vi "SimulatoreStep.vi"() -> ()   [LabVIEW 2019]
doc: "Simulatore Step dei Test:\n\n1. Seleziona la postazione con la data di partenza (opzionale)\n2. Seleziona il Test che vuoi eseguire\n3. Avvia la simulazione e verifica il successo degli Step"
uses:
  ByteGSAPIBase/ByteGSAPIBase.lvclass
  TypeDef/StepSimulationInfo.ctl
  TypeDef/ProcessStatus.ctl
  TypeDef/SimulatoreStates.ctl
  ByteGSAPIBase/TypeDef/Step.ctl
  ByteGSAPIBase/TypeDef/Asset.ctl
  ByteGSAPIBase/TypeDef/Test.ctl
  <vilib>/numeric/Random Number (Range) U64.vi
  <vilib>/numeric/sub_Random U32.vi
panel:
  out "Title":string
  out "Status Control":T2
  out "Waveform Chart":cluster{"Time Elapsed":dbl, dbl}(graph)
  out "Step Info List":T3[](array[typedef])
  in  "Step simulation":bool
  out "Infos":string
  in  "Inizia Test":bool
  in  "Select Test":i32(ring) items=["T0014 - Endurance test"=54, "T0011 - Endurance test 19/02/2025"=51, "T0010 - Endurance test 19/02/2025"=50, "T0009 - Endurance test 19/02/2025"=49, "T0006 - Endurance Test"=46, "T0007 - Endurance Test"=47, "T0012 - Endurance test"=52, "T0013 - Endurance test"=53, "T0005 - Endurance Test"=45, "T0015 - Endurance test"=55, "T0008 - Endurance test 19/02/2025"=48, "T0016 - Endurance test"=56]
  in  "ByteGSAPIBase in":refnum<class "ByteGSAPIBase.lvclass">
  in  "Exit":bool
  in  "Home":bool
  in  "Ottieni Test Per Postazione":bool
  in  "Starting Date":timestamp format="%<%x>T"
  in  "Workstation":u16(ring) items=["Sala gialla", "POST 1"]
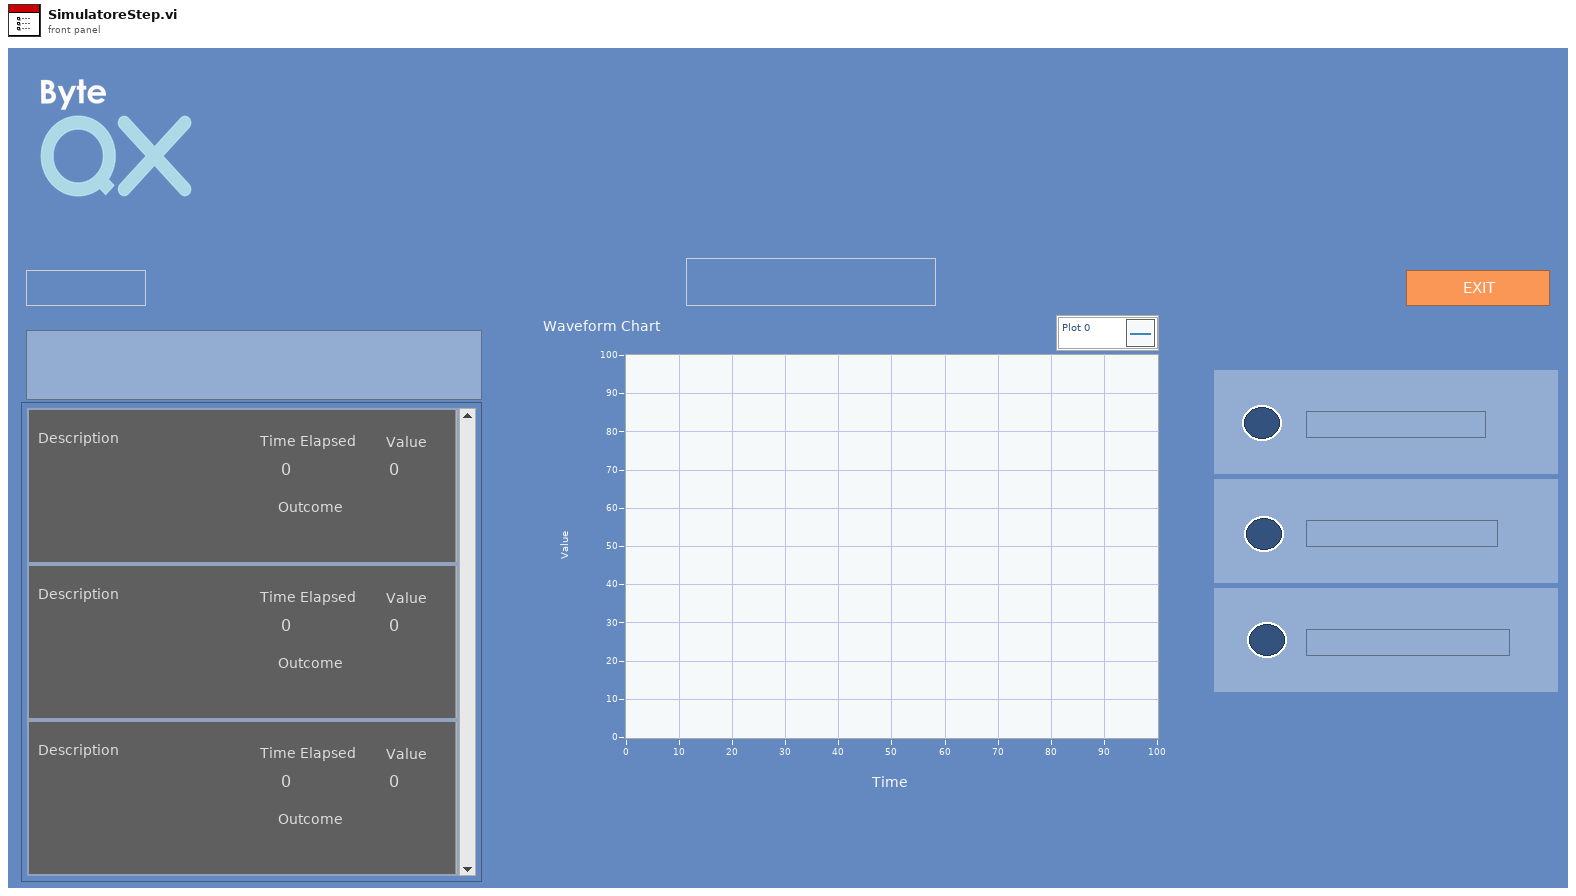
[diagram p1: front panel]
types:
  T1 = typedef "ProcessStatus.ctl" = cluster{"Active":bool, "Process":string}
  T2 = cluster{"Cluster":T1, "Cluster 2":T1, "Cluster 3":T1}
  T3 = typedef "StepSimulationInfo.ctl" = cluster{"Description":string, "Value":dbl, "Outcome":string, "Time Elapsed":dbl, "id":dbl, "Color Box":u32}
  T4 = typedef "SimulatoreStates.ctl" = enum16{"Initialize", "Idle", "GetLimsTestsForBench", "GetLimsTestSteps", "Simulation Start", "WaitForLigths"}
  T5 = typedef "ByteQXWebAPI.lvlib/ByteGSAPIBase.lvclass/Test.ctl" = cluster{"titolo":string, "descrizione":string, "statoprova":string, "assets":T6[], "id":i32, "data_apertura_prova":timestamp, "slug":string}
  T6 = typedef "ByteQXWebAPI.lvlib/ByteGSAPIBase.lvclass/Asset.ctl" = cluster{"descrizione":string, "slug":string, "id":i32}
  T7 = typedef "ByteQXWebAPI.lvlib/ByteGSAPIBase.lvclass/Step.ctl" = cluster{"id":i32, "descrizione":string, "prova":cluster{"slug":string}, "assets":T6[], "criterio_accettazione":string, "valore_criterio_accettazione_max":dbl, "valore_criterio_accettazione_min":dbl, "udm_criterio_accettazione":string, "duration_prova":string, "udm_duration_prova":string, "valore_prova":dbl, "ordine":i32, "user":i32, "link_automation":string, "instruction_automation":string, "data_completamento_checklist":timestamp, "outcome":bool, "step_type":string, "channels":string[]}
  T8 = cluster{"ByteGSAPIBase in":refnum<class "ByteGSAPIBase.lvclass">, "Array dei Test":T5[], "Steps Array":T7[], "Step Info List":T3[], "index":i32, "Previus":T4, "Infos":string, "State":T4, "Status Control":cluster{"Cluster":T1, "Cluster 2":T1, "Cluster 3":T1}, "light position":i32}
  T9 = cluster{"Workstation":refnum<vi>, "Starting Date":refnum<vi>, "Ottieni Test Per Postazione":refnum<vi>, "Infos":refnum<vi>, "Inizia Test":refnum<vi>, "Select Test":refnum<vi>, "Step Info List":refnum<vi>, "Step simulation":refnum<vi>, "Waveform Chart":refnum<vi>, "Status Control":refnum<vi>, "Title":refnum<vi>}
  T10 = enum8{"Enabled", "Disabled", "Disabled and Grayed Out"}
  T11 = cluster{"Workstation":u16, "Starting Date":timestamp, "Select Test":i32}
  T12 = typedef "ByteQXWebAPI.lvlib/ByteGSAPIBase.lvclass/UpdateLimsTestStepData.ctl" = cluster{"outcome":bool, "data_completamento_checklist":timestamp, "udm_duration_prova":string, "valore_prova":dbl, "link_automation":string, "instruction_automation":string, "duration_prova":string}
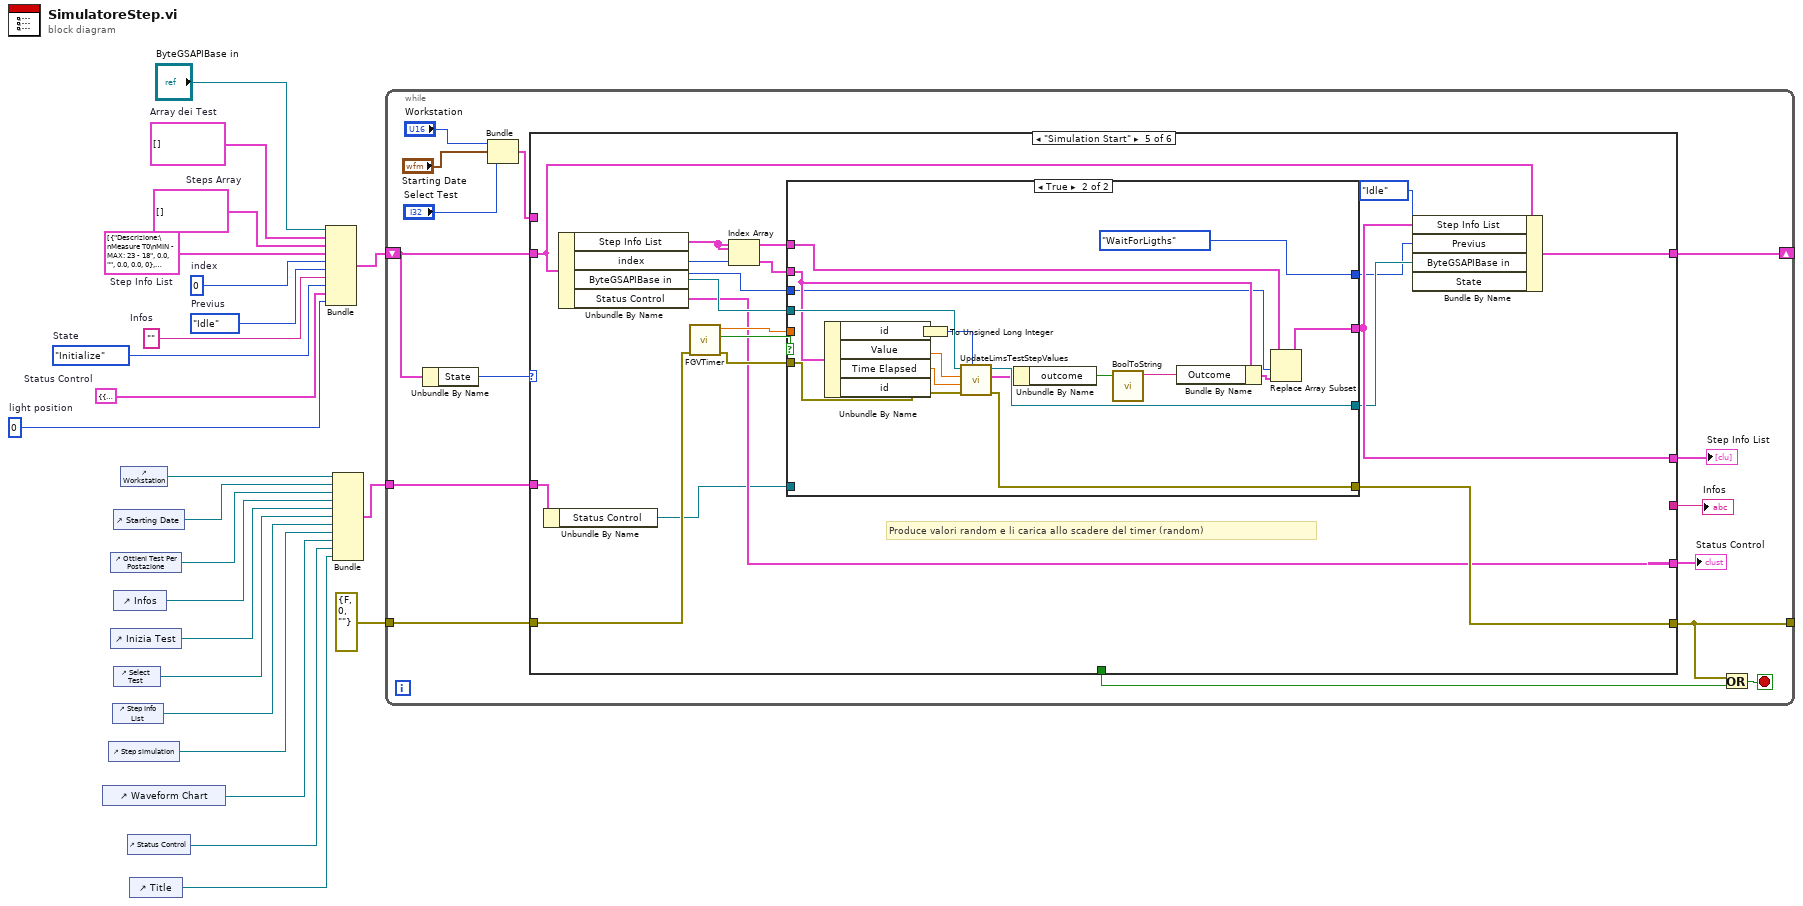
[diagram p0: block diagram]
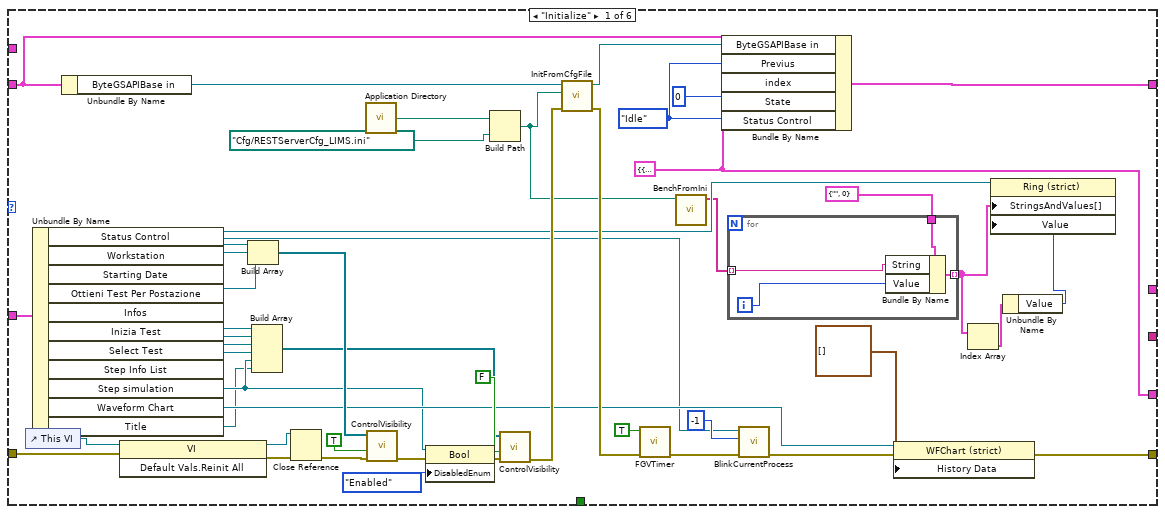
[diagram p2: hidden frame]
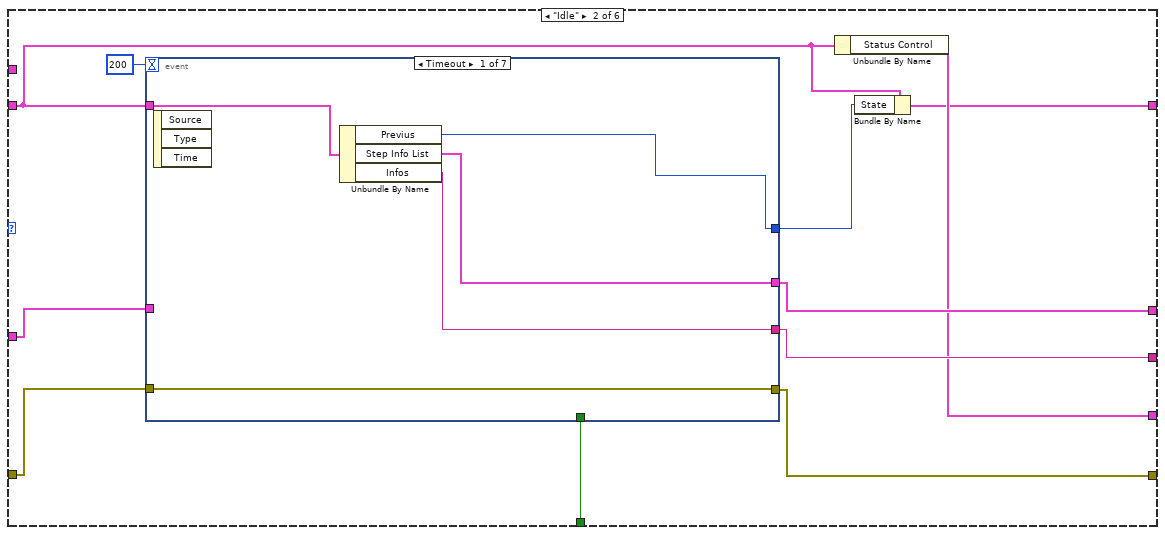
[diagram p3: hidden frame]
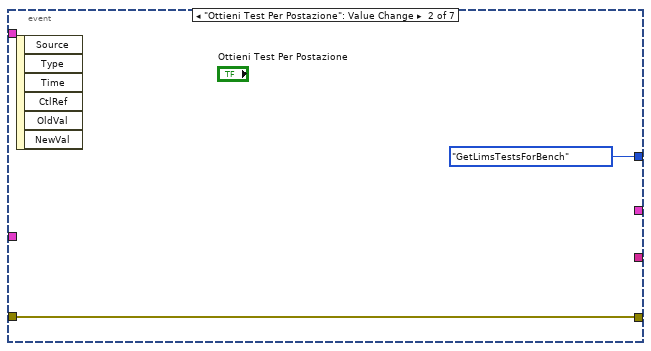
[diagram p4: hidden frame]
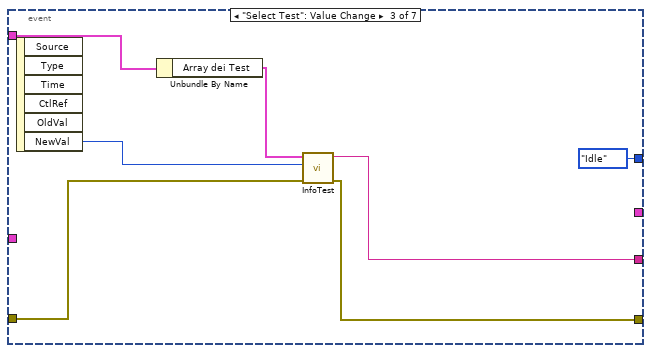
[diagram p5: hidden frame]
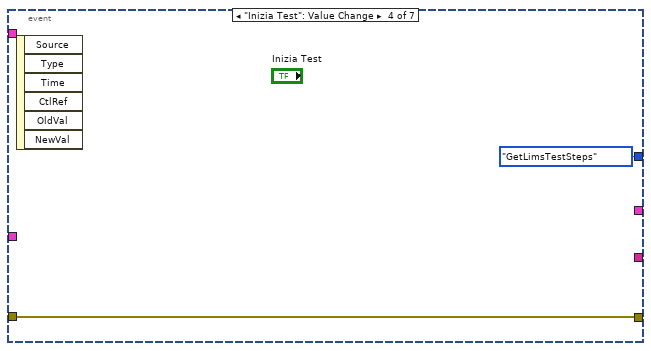
[diagram p6: hidden frame]
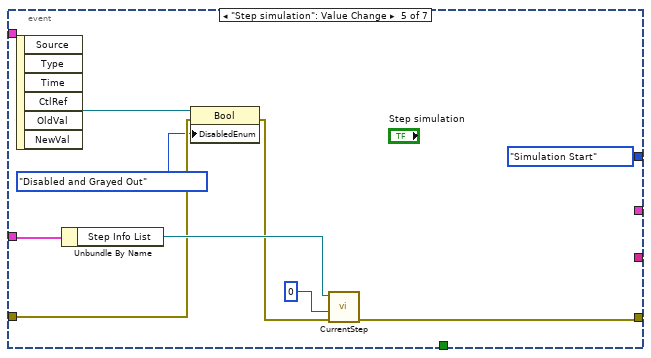
[diagram p7: hidden frame]
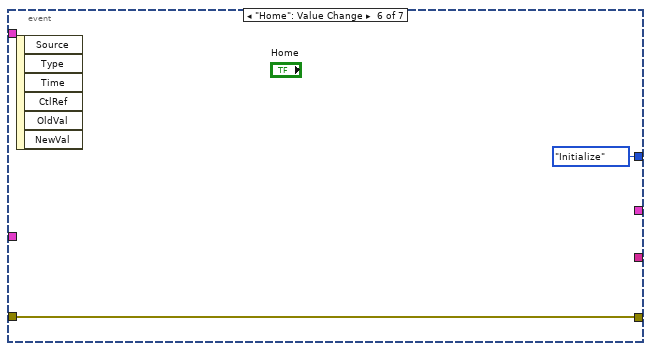
[diagram p8: hidden frame]
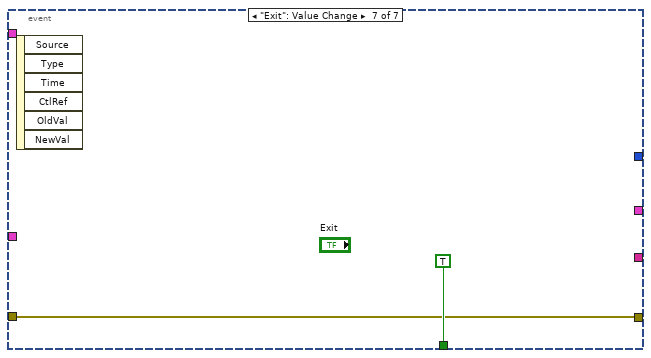
[diagram p9: hidden frame]
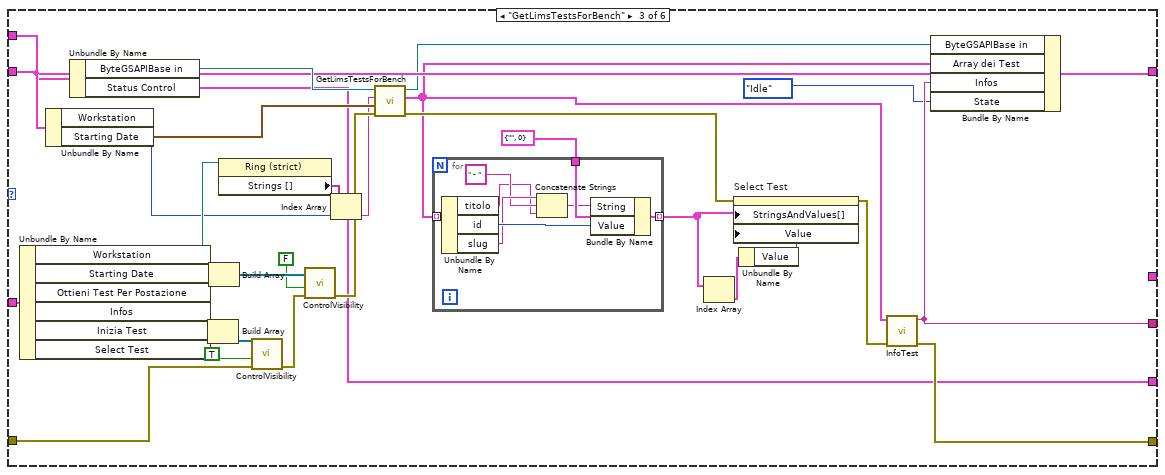
[diagram p10: hidden frame]
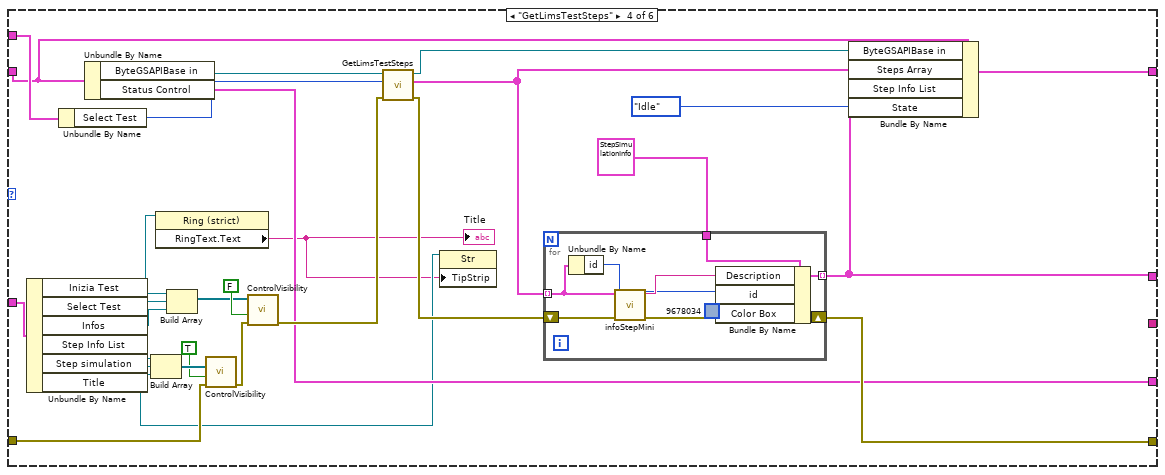
[diagram p11: hidden frame]
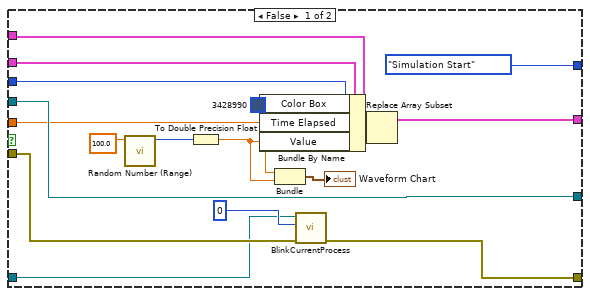
[diagram p12: hidden frame]
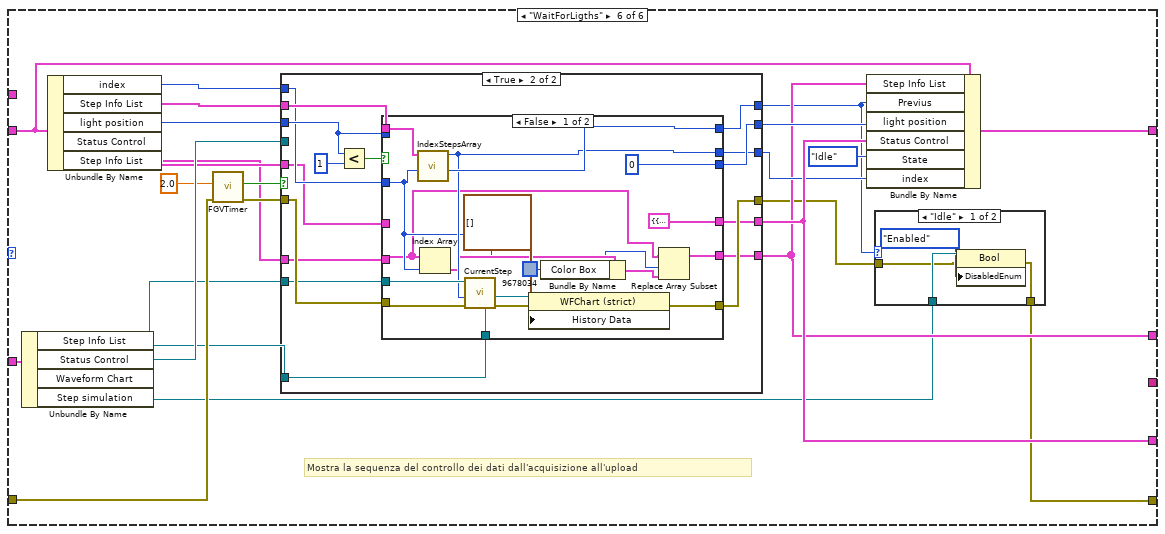
[diagram p13: hidden frame]
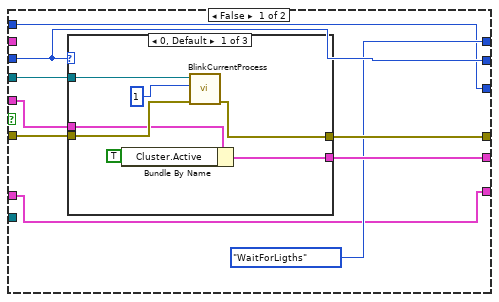
[diagram p15: hidden frame]
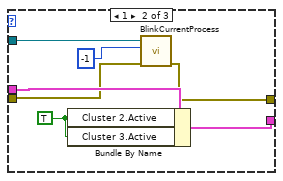
[diagram p16: hidden frame]
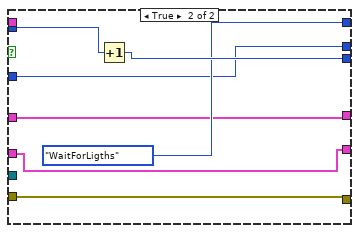
[diagram p18: hidden frame]
diagram:
  w5 = 0  # light position
  w6 = T2 {"Cluster"={"Active"=FALSE, "Process"="Acquisizione Dati"}, "Cluster 2"={"Active"=FALSE, "Process"="Upload Dati"}, "Cluster 3"={"Active"=FALSE, "Process"="Upload Completato"}}  # Status Control
  w9 = ""  # Infos
  w10 = SimulatoreStates."Idle"  # Previus
  w11 = 0  # index
  w12 = T3[] [{"Description"="Descrizione:\nMeasure T0\nMIN - MAX: 23 - 18", "Value"=0.0, "Outcome"="", "Time Elapsed"=0.0, "id"=0.0, "Color Box"=0}, {"Description"="Descrizione:\nSet Nominsl Torque\nMIN - MAX: 1 - -1", "Value"=0.0, "Outcome"="", "Time Elapsed"=0.0, "id"=0.0, "Color Box"=0}, {"Description"="Descrizione:\nVibrazione X,Y,Z\nMIN - MAX: 0 - 0", "Value"=0.0, "Outcome"="", "Time Elapsed"=0.0, "id"=0.0, "Color Box"=0}, {"Description"="Descrizione:\nPlace Motor on the bench. Plug wires on terminal block.\nMIN - MAX: 0 - 0", "Value"=0.0, "Outcome"="", "Time Elapsed"=0.0, "id"=0.0, "Color Box"=0}, {"Description"="Descrizione:\nMeasure R01\nMIN - MAX: 0 - 0", "Value"=0.0, "Outcome"="", "Time Elapsed"=0.0, "id"=0.0, "Color Box"=0}, {"Description"="Descrizione:\nMeasure R02\nMIN - MAX: 0 - 0", "Value"=0.0, "Outcome"="", "Time Elapsed"=0.0, "id"=0.0, "Color Box"=0}]  # Step Info List
  w19 = T5[] []  # Array dei Test
  w18 = T7[] []  # Steps Array
  w8 = SimulatoreStates."Initialize"  # State
  n1 = control-ref of="Waveform Chart"() -> (w3:refnum<vi>)
  n2 = control-ref of="Step simulation"() -> (w13:refnum<vi>)
  n3 = control-ref of="Ottieni Test Per Postazione"() -> (w22:refnum<vi>)
  n4 = control-ref of="Inizia Test"() -> (w15:refnum<vi>)
  n5 = control-ref of="Step Info List"() -> (w4:refnum<vi>)
  n6 = control-ref of="Starting Date"() -> (w23:refnum<vi>)
  n7 = control-ref of="Infos"() -> (w16:refnum<vi>)
  n8 = control-ref of="Select Test"() -> (w14:refnum<vi>)
  n9 = control-ref of="Workstation"() -> (w24:refnum<vi>)
  n10 = control-ref of="Status Control"() -> (w2:refnum<vi>)
  n11 = control-ref of="Title"() -> (w1:refnum<vi>)
  n12 = Bundle("ByteGSAPIBase in"="ByteGSAPIBase in", "Array dei Test"=w19, "Steps Array"=w18, "Step Info List"=w12, "index"=w11, "Previus"=w10, "Infos"=w9, "State"=w8, "Status Control"=w6, "light position"=w5) -> (w17:T8)  [unwired: 1 in]
  n13 = Bundle("Workstation"=w24, "Starting Date"=w23, "Ottieni Test Per Postazione"=w22, "Infos"=w16, "Inizia Test"=w15, "Select Test"=w14, "Step Info List"=w4, "Step simulation"=w13, "Waveform Chart"=w3, "Status Control"=w2, "Title"=w1) -> (w21:T9)  [unwired: 1 in]
  n14 = while {
    tunnel: w21 -> [w35]
    shift-right: [w34] -> _
    shift-left: w17 -> [w28]
    tunnel: errorcluster {"status"=FALSE, "code"=0, "source"=""} ("error in (no error)") -> [w39]
    tunnel: [w31] -> _
    stop <- w30 stop-if-true
    n15 = Unbundle By Name(w28) -> ("State"=w27:T4)
    n16 = Bundle("Workstation"="Workstation", "Starting Date"="Starting Date", "Select Test"="Select Test") -> (w36:T11)  [unwired: 1 in]
    n17 = case shown="\"Simulation Start\"" w27 {
      tunnel: w39 -> [w85 w101 w158 w184 w225 w280]
      tunnel: w36 -> [_ _ w163 w200 _ _]
      tunnel: w35 -> [w82 w95 w154 w194 w212 w282]
      tunnel: [w60 w99 w145 w188 w214 w262] -> w31
      tunnel: w28 -> [w73 w92 w162 w197 w222 w277]
      tunnel: [w72 w91 w160 w196 w218 w276] -> w34
      tunnel: [_ w100 w140 _ _ _] -> w32
      tunnel: [_ w97 _ w180 w219 w266] -> w26
      tunnel: [_ w96 _ _ _ _] -> w29
      tunnel: [w54 w93 w137 w177 w210 w274] -> w25
      frame "Initialize" {
        w54 = T2 {"Cluster"={"Active"=FALSE, "Process"="DATA AQUISITION"}, "Cluster 2"={"Active"=FALSE, "Process"="DATA UPLOAD"}, "Cluster 3"={"Active"=FALSE, "Process"="LOADING NEXT STEP"}} ("Status Control")
        w61 = SimulatoreStates."Idle"
        n18 = control-ref of="This VI"() -> (w86:refnum<vi>)
        n19 = Unbundle By Name(w82) -> ("Status Control"=w53:refnum<vi>, "Workstation"=w45:refnum<vi>, "Starting Date"=w81:refnum<vi>, "Ottieni Test Per Postazione"=w80:refnum<vi>, "Infos"=w69:refnum<vi>, "Inizia Test"=w68:refnum<vi>, "Select Test"=w67:refnum<vi>, "Step Info List"=w65:refnum<vi>, "Step simulation"=w50:refnum<vi>, "Waveform Chart"=w59:refnum<vi>, "Title"=w48:refnum<vi>)
        n20 = Unbundle By Name(w73) -> ("ByteGSAPIBase in"=w74:refnum<class "ByteGSAPIBase.lvclass">)
        n21 = invoke class="VI" method="Default Vals.Reinit All"(reference=w86, error in=w85) -> (reference out=w84:refnum<vi>, error out=w83:errorcluster)  [unwired: 1 in, 1 out]
        n22 = Build Array(w45, w81, w80) -> (w79:refnum<vi>[])
        n23 = Build Array(w69, w68, w67, w65, w50, w48) -> (w66:refnum<vi>[])
        n24 = Close Reference(reference=w84, error in (no error)=w83) -> (error out=w78:errorcluster)
        n25 = call <vilib>:"Application Directory.vi"() -> ("Application Directory"=w76:path)
        n26 = call "ControlVisibility.vi"("error in (no error)"=w78, "Visible"=TRUE, "Controls"=w79) -> ("error out"=w52:errorcluster)  [unwired: 8 in]
        n27 = property class="Bool"(reference=w50, error in=w52, "DisabledEnum"=T10."Enabled" ("Disabled")) -> (error out=w51:errorcluster)  [unwired: 1 out]
        n28 = Build Path(base path=w76, name or relative path=path "Cfg/RESTServerCfg_LIMS.ini") -> (appended path=w46:path)
        n29 = call "ControlVisibility.vi"("error in (no error)"=w51, "Visible"=FALSE, "Controls"=w66) -> ("error out"=w71:errorcluster)  [unwired: 8 in]
        n30 = call-dynamic "InitFromCfgFile.vi"("error in (no error)"=w71, "configuration file path"=w46, "ByteGSAPIBase in"=w74) -> ("error out"=w64:errorcluster, "ByteGSAPIBase out"=w75:refnum<class "ByteGSAPIBase.lvclass">)  [unwired: 7 in]
        n31 = call "FGVTimer.vi"("error in"=w64, "Reset"=TRUE) -> ("error out"=w57:errorcluster)  [unwired: 7 in, 2 out]
        n32 = call "BenchFromIni.vi"("configuration file path"=w46) -> ("Array"=w44:string[])  [unwired: 9 in, 1 out]
        n33 = Bundle By Name(cluster=w73, "ByteGSAPIBase in"=w75, "Previus"=w61, "index"=0, "State"=w61, "Status Control"=w54) -> (w72:T8)
        n34 = for {
          tunnel: [w90] -> w41 mode=indexing
          tunnel: w44 -> [w89] mode=indexing
          tunnel: cluster{"String":string, "Value":u16} {"String"="", "Value"=0} ("Cluster") -> [w87]
          i -> [w88]
          n35 = Bundle By Name(cluster=w87, "String"=w89, "Value"=w88) -> (w90:cluster{"String":string, "Value":u16})
        }
        n36 = call "BlinkCurrentProcess.vi"("error in (no error)"=w57, "index"=-1, "Status Control"=w53) -> ("error out"=w56:errorcluster)  [unwired: 8 in]
        n37 = property class="WFChart (strict)"(reference=w59, error in=w56, "History Data"=cluster{"Time Elapsed":dbl, dbl}[] []) -> (error out=w60:errorcluster)  [unwired: 1 out]
        n38 = Index Array(array=w41) -> (element=w42:cluster{"String":string, "Value":u16})  [unwired: 1 in]
        n39 = Unbundle By Name(w42) -> ("Value"=w40:u16)
        n40 = property class="Ring (strict)"(reference=w45, "StringsAndValues[]"=w41, "Value"=w40) -> ()  [unwired: 1 in, 2 out]
      }
      frame "Idle" {
        n41 = event shown="[0] Timeout" {
          selector: _ -> [_ _ _ _ _ _ _]
          dyn-events: _ -> [_ _ _ _ _ _ _]
          timeout: 200 -> [_ _ _ _ _ _ _]
          tunnel: [w102 SimulatoreStates."GetLimsTestsForBench" SimulatoreStates."Idle" SimulatoreStates."GetLimsTestSteps" SimulatoreStates."Simulation Start" SimulatoreStates."Initialize" _] -> w94
          tunnel: [w104 _ w114 _ _ _ _] -> w100
          tunnel: w101 -> [w103 w107 w113 w116 w120 w127 w129]
          tunnel: [w103 w107 w112 w116 w124 w127 w129] -> w99
          tunnel: w92 -> [w106 _ w111 _ _ _ _]
          tunnel: [w105 _ _ _ _ _ _] -> w97
          tunnel: [_ _ _ _ _ _ TRUE] -> w96
          tunnel: w95 -> [_ _ _ _ w125 _ _]
          event Timeout {
            n42 = event-data() -> ()  [unwired: 1 in, 3 out]
            n43 = Unbundle By Name(w106) -> ("Previus"=w102:T4, "Step Info List"=w105:T3[], "Infos"=w104:string)
          }
          event "Ottieni Test Per Postazione": Value Change {
            n44 = event-data() -> ()  [unwired: 1 in, 6 out]
          }
          event "Select Test": Value Change {
            n45 = event-data() -> ("NewVal"=w110:i32)  [unwired: 1 in, 5 out]
            n46 = Unbundle By Name(w111) -> ("Array dei Test"=w109:T5[])
            n47 = call "InfoTest.vi"("error in"=w113, "Seleziona Test"=w110, "TestForBenchArray"=w109) -> ("error out"=w112:errorcluster, "Info Test"=w114:string)  [unwired: 7 in]
          }
          event "Inizia Test": Value Change {
            n48 = event-data() -> ()  [unwired: 1 in, 6 out]
          }
          event "Step simulation": Value Change {
            n49 = event-data() -> ("CtlRef"=w121:refnum<vi>)  [unwired: 1 in, 5 out]
            n50 = Unbundle By Name(w125) -> ("Step Info List"=w122:refnum<vi>)
            n51 = property class="Bool"(reference=w121, error in=w120, "DisabledEnum"=T10."Disabled and Grayed Out" ("Disabled")) -> (error out=w119:errorcluster)  [unwired: 1 out]
            n52 = call "CurrentStep.vi"("error in (no error)"=w119, "index"=0, "Array in"=w122) -> ("error out"=w124:errorcluster)  [unwired: 8 in]
          }
          event "Home": Value Change {
            n53 = event-data() -> ()  [unwired: 1 in, 6 out]
          }
          event "Exit": Value Change {
            n54 = event-data() -> ()  [unwired: 1 in, 6 out]
          }
        }
        n55 = Unbundle By Name(w92) -> ("Status Control"=w93:T2)
        n56 = Bundle By Name(cluster=w92, "State"=w94) -> (w91:T8)
      }
      frame "GetLimsTestsForBench" {
        n57 = Unbundle By Name(w154) -> ("Workstation"=w134:refnum<vi>, "Starting Date"=w153:refnum<vi>, "Ottieni Test Per Postazione"=w152:refnum<vi>, "Infos"=w151:refnum<vi>, "Inizia Test"=w150:refnum<vi>, "Select Test"=w149:refnum<vi>)
        n58 = Unbundle By Name(w163) -> ("Workstation"=w132:u16, "Starting Date"=w139:timestamp)
        n59 = Unbundle By Name(w162) -> ("ByteGSAPIBase in"=w164:refnum<class "ByteGSAPIBase.lvclass">, "Status Control"=w137:T2)
        n60 = Build Array(w151, w150, w149) -> (w143:refnum<vi>[])
        n61 = Build Array(w134, w153, w152) -> (w144:refnum<vi>[])
        n62 = property class="Ring (strict)"(reference=w134) -> ("Strings []"=w133:string[])  [unwired: 1 in, 2 out]
        n63 = call "ControlVisibility.vi"("error in (no error)"=w158, "Visible"=TRUE, "Controls"=w143) -> ("error out"=w148:errorcluster)  [unwired: 8 in]
        n64 = call "ControlVisibility.vi"("error in (no error)"=w148, "Visible"=FALSE, "Controls"=w144) -> ("error out"=w147:errorcluster)  [unwired: 8 in]
        n65 = Index Array(array=w133, index=w132) -> (element=w131:string)
        n66 = call-dynamic "GetLimsTestsForBench.vi"("error in (no error)"=w147, "creation date"=w139, "workbench"=w131, "ByteGSAPIBase in"=w164) -> ("error out"=w136:errorcluster, "list of tests"=w135:T5[], "ByteGSAPIBase out"=w161:refnum<class "ByteGSAPIBase.lvclass">)  [unwired: 5 in]
        n67 = for {
          tunnel: [w171] -> w157 mode=indexing
          tunnel: cluster{"String":string, "Value":u16} {"String"="", "Value"=0} ("Cluster") -> [w170]
          tunnel: w135 -> [w169] mode=indexing
          n68 = Unbundle By Name(w169) -> ("titolo"=w166:string, "id"=w172:i32, "slug"=w168:string)
          n69 = Concatenate Strings(w168, " - " ("string"), w166) -> (w165:string)
          n70 = Bundle By Name(cluster=w170, "String"=w165, "Value"=w172) -> (w171:cluster{"String":string, "Value":u16})
        }
        n71 = Index Array(array=w157) -> (element=w156:cluster{"String":string, "Value":u16})  [unwired: 1 in]
        n72 = Unbundle By Name(w156) -> ("Value"=w155:u16)
        n73 = property on="Select Test" class="Ring (strict)"(error in=w136, "StringsAndValues[]"=w157, "Value"=w155) -> (error out=w146:errorcluster)  [unwired: 1 in, 1 out]
        n74 = call "InfoTest.vi"("error in"=w146, "TestForBenchArray"=w135) -> ("error out"=w145:errorcluster, "Info Test"=w140:string)  [unwired: 8 in]
        n75 = Bundle By Name(cluster=w162, "ByteGSAPIBase in"=w161, "Array dei Test"=w135, "Infos"=w140, "State"=SimulatoreStates."Idle") -> (w160:T8)
      }
      frame "GetLimsTestSteps" {
        n76 = Unbundle By Name(w194) -> ("Inizia Test"=w193:refnum<vi>, "Select Test"=w176:refnum<vi>, "Infos"=w187:refnum<vi>, "Step Info List"=w186:refnum<vi>, "Step simulation"=w181:refnum<vi>, "Title"=w174:refnum<vi>)
        n77 = Unbundle By Name(w200) -> ("Select Test"=w175:i32)
        n78 = Unbundle By Name(w197) -> ("ByteGSAPIBase in"=w199:refnum<class "ByteGSAPIBase.lvclass">, "Status Control"=w177:T2)
        n79 = Build Array(w186, w181, w174) -> (w185:refnum<vi>[])
        n80 = property class="Ring (strict)"(reference=w176) -> ("RingText.Text"=w173:string)  [unwired: 1 in, 2 out]
        "Title" <- w173
        n81 = Build Array(w193, w176, w187) -> (w192:refnum<vi>[])
        n82 = call "ControlVisibility.vi"("error in (no error)"=w184, "Visible"=TRUE, "Controls"=w185) -> ("error out"=w183:errorcluster)  [unwired: 8 in]
        n83 = call "ControlVisibility.vi"("error in (no error)"=w183, "Visible"=FALSE, "Controls"=w192) -> ("error out"=w191:errorcluster)  [unwired: 8 in]
        n84 = call-dynamic "GetLimsTestSteps.vi"("error in (no error)"=w191, "test-id"=w175, "ByteGSAPIBase in"=w199) -> ("error out"=w189:errorcluster, "list of steps"=w190:T7[], "ByteGSAPIBase out"=w198:refnum<class "ByteGSAPIBase.lvclass">)  [unwired: 6 in]
        n85 = property class="Str"(reference=w174, "TipStrip"=w173) -> ()  [unwired: 1 in, 2 out]
        n86 = for {
          tunnel: w190 -> [w203] mode=indexing
          shift-right: [w207] -> w188
          shift-left: w189 -> [w208]
          tunnel: T3 {"Description"="Descrizione:\nMeasure T0\nMIN - MAX: 23 - 18", "Value"=0.0, "Outcome"="", "Time Elapsed"=0.0, "id"=0.0, "Color Box"=0} ("Cluster") -> [w206]
          tunnel: [w204] -> w180 mode=indexing
          n87 = Unbundle By Name(w203) -> ("id"=w202:i32)
          n88 = call "infoStepMini.vi"("error in (no error)"=w208, "StepList"=w203) -> ("error out"=w207:errorcluster, "Info Test"=w205:string)  [unwired: 8 in]
          n89 = Bundle By Name(cluster=w206, "Description"=w205, "id"=w202, "Color Box"=u32 9678034) -> (w204:T3)
        }
        n90 = Bundle By Name(cluster=w197, "ByteGSAPIBase in"=w198, "Steps Array"=w190, "Step Info List"=w180, "State"=SimulatoreStates."Idle") -> (w196:T8)
      }
      frame "Simulation Start" {
        # "Produce valori random e li carica allo scadere del timer (random)"
        n91 = Unbundle By Name(w212) -> ("Status Control"=w209:refnum<vi>)
        n92 = Unbundle By Name(w222) -> ("Step Info List"=w221:T3[], "index"=w220:i32, "ByteGSAPIBase in"=w217:refnum<class "ByteGSAPIBase.lvclass">, "Status Control"=w210:T2)
        n93 = call "FGVTimer.vi"("error in"=w225) -> ("error out"=w216:errorcluster, "Elapsed?"=w226:bool, "Time Elapsed"=w223:dbl)  [unwired: 8 in]
        n94 = Index Array(array=w221, index=w220) -> (element=w224:T3)
        n95 = case shown="True" w226 {
          tunnel: w224 -> [w243 w257]
          tunnel: w223 -> [w234 _]
          tunnel: w221 -> [w241 w251]
          tunnel: w220 -> [w235 w252]
          tunnel: [w239 w260] -> w219
          tunnel: w217 -> [w238 w258]
          tunnel: w216 -> [w232 w248]
          tunnel: [w238 w254] -> w215
          tunnel: [w231 w246] -> w214
          tunnel: [SimulatoreStates."Simulation Start" ("Previus") SimulatoreStates."WaitForLigths" ("Previus")] -> w213
          tunnel: w209 -> [w227 _]
          frame False {
            n96 = call-poly <vilib>:"Random Number (Range).vi"("upper bound (100)"=100.0) -> ("number"=w236:u64)  [unwired: 10 in]
            n97 = To Double Precision Float(number=w236) -> (double precision float=w233:dbl)
            n98 = Bundle By Name(cluster=w243, "Color Box"=u32 3428990, "Time Elapsed"=w234, "Value"=w233) -> (w240:T3)
            n99 = Bundle("Time Elapsed"=w234, w233) -> (→"Waveform Chart":cluster{"Time Elapsed":dbl, dbl})  [unwired: 1 in]
            n100 = call "BlinkCurrentProcess.vi"("error in (no error)"=w232, "index"=0, "Status Control"=w227) -> ("error out"=w231:errorcluster)  [unwired: 8 in]
            n101 = Replace Array Subset(array=w241, new element=w240, index=w235) -> (w239:T3[])
          }
          frame True {
            n102 = Unbundle By Name(w257) -> ("id"=w245:dbl, "Value"=w256:dbl, "Time Elapsed"=w255:dbl)  [unwired: 1 out]
            n103 = To Unsigned Long Integer(number=w245) -> (unsigned 32bit integer=w244:u32)
            n104 = call-dynamic "UpdateLimsTestStepValues.vi"("step-id"=w244, "error in (no error)"=w248, "duration hours"=w255, "value"=w256, "ByteGSAPIBase in"=w258) -> ("error out"=w246:errorcluster, "step result"=w253:T12, "ByteGSAPIBase out"=w254:refnum<class "ByteGSAPIBase.lvclass">)  [unwired: 4 in]
            n105 = Unbundle By Name(w253) -> ("outcome"=w249:bool)
            n106 = call "BoolToString.vi"("outcome"=w249) -> ("String"=w250:string)  [unwired: 10 in]
            n107 = Bundle By Name(cluster=w257, "Outcome"=w250) -> (w259:T3)
            n108 = Replace Array Subset(array=w251, new element=w259, index=w252) -> (w260:T3[])
          }
        }
        n109 = Bundle By Name(cluster=w222, "Step Info List"=w219, "Previus"=w213, "ByteGSAPIBase in"=w215, "State"=SimulatoreStates."Idle") -> (w218:T8)
      }
      frame "WaitForLigths" {
        # "Mostra la sequenza del controllo dei dati dall'acquisizione all'upload"
        n110 = Unbundle By Name(w282) -> ("Step Info List"=w269:refnum<vi>, "Status Control"=w281:refnum<vi>, "Waveform Chart"=w268:refnum<vi>, "Step simulation"=w264:refnum<vi>)
        n111 = Unbundle By Name(w277) -> ("index"=w271:i32, "Step Info List"=w272:T3[], "light position"=w283:i32, "Status Control"=w278:T2, "Step Info List"=w267:T3[])
        n112 = call "FGVTimer.vi"("error in"=w280, "set timer"=2.0) -> ("error out"=w279:errorcluster, "Elapsed?"=w284:bool)  [unwired: 7 in, 1 out]
        n113 = case shown="True" w284 {
          tunnel: w283 -> [w293 w328]
          tunnel: w281 -> [w298 _]
          tunnel: w279 -> [w297 w322]
          tunnel: w278 -> [w296 w317]
          tunnel: [w295 w318] -> w274
          tunnel: [w294 w320] -> w263
          tunnel: [w293 w327] -> w273
          tunnel: [SimulatoreStates."WaitForLigths" ("Previus") w326] -> w265
          tunnel: w272 -> [_ w325]
          tunnel: w271 -> [w291 w324]
          tunnel: [w291 w323] -> w270
          tunnel: w269 -> [_ w321]
          tunnel: w268 -> [_ w319]
          tunnel: w267 -> [w290 w316]
          tunnel: [w290 w315] -> w266
          frame False {
            n114 = case shown="0, Default" w293 {
              tunnel: w298 -> [w299 w306 _]
              tunnel: w297 -> [w304 w310 w313]
              tunnel: w296 -> [w302 w311 w314]
              tunnel: [w301 w309 w314] -> w295
              tunnel: [w300 w308 w313] -> w294
              frame 0, Default {
                n115 = Bundle By Name(cluster=w302, "Cluster.Active"=TRUE) -> (w301:T2)
                n116 = call "BlinkCurrentProcess.vi"("error in (no error)"=w304, "index"=1, "Status Control"=w299) -> ("error out"=w300:errorcluster)  [unwired: 8 in]
              }
              frame 1 {
                w307 = TRUE ("Cluster.Active")
                n117 = Bundle By Name(cluster=w311, "Cluster 2.Active"=w307, "Cluster 3.Active"=w307) -> (w309:T2)
                n118 = call "BlinkCurrentProcess.vi"("error in (no error)"=w310, "index"=-1, "Status Control"=w306) -> ("error out"=w308:errorcluster)  [unwired: 8 in]
              }
              frame 2 {
              }
            }
          }
          frame True {
            n119 = Less?(x=w328, y=1) -> (x < y?=w329:bool)
            n120 = case shown="False" w329 {
              tunnel: w328 -> [_ w354]
              tunnel: [0 w353] -> w327
              tunnel: [w346 SimulatoreStates."WaitForLigths" ("Previus")] -> w326
              tunnel: w325 -> [w345 _]
              tunnel: w324 -> [w334 w351]
              tunnel: [w338 w351] -> w323
              tunnel: w322 -> [w344 w350]
              tunnel: w321 -> [w343 _]
              tunnel: [w340 w350] -> w320
              tunnel: w319 -> [w339 _]
              tunnel: [T2 {"Cluster"={"Active"=FALSE, "Process"="DATA AQUISITION"}, "Cluster 2"={"Active"=FALSE, "Process"="DATA UPLOAD"}, "Cluster 3"={"Active"=FALSE, "Process"="LOADING NEXT STEP"}} ("Status Control") w349] -> w318
              tunnel: w317 -> [_ w349]
              tunnel: w316 -> [w333 w348]
              tunnel: [w332 w348] -> w315
              frame False {
                n121 = call "IndexStepsArray.vi"("index"=w334, "Steps Array"=w345) -> ("Previus"=w346:T4, "Index out"=w338:i32)  [unwired: 8 in]
                n122 = Index Array(array=w333, index=w334) -> (element=w337:T3)
                n123 = call "CurrentStep.vi"("error in (no error)"=w344, "index"=w338, "Array in"=w343) -> ("error out"=w342:errorcluster)  [unwired: 8 in]
                n124 = property class="WFChart (strict)"(reference=w339, error in=w342, "History Data"=cluster{"Time Elapsed":dbl, dbl}[] []) -> (error out=w340:errorcluster)  [unwired: 1 out]
                n125 = Bundle By Name(cluster=w337, "Color Box"=u32 9678034) -> (w335:T3)
                n126 = Replace Array Subset(array=w333, new element=w335, index=w334) -> (w332:T3[])
              }
              frame True {
                n127 = Increment(x=w354) -> (x+1=w353:i32)
              }
            }
          }
        }
        n128 = Bundle By Name(cluster=w277, "Step Info List"=w266, "Previus"=w265, "light position"=w273, "Status Control"=w274, "State"=SimulatoreStates."Idle", "index"=w270) -> (w276:T8)
        n129 = case shown="\"Idle\"" w265 {
          tunnel: w264 -> [w288 _]
          tunnel: w263 -> [w286 w289]
          tunnel: [w285 w289] -> w262
          frame "Idle" {
            n130 = property class="Bool"(reference=w288, error in=w286, "DisabledEnum"=T10."Enabled" ("Disabled")) -> (error out=w285:errorcluster)  [unwired: 1 out]
          }
          frame Default {
          }
        }
      }
    }
    "Infos" <- w32
    "Step Info List" <- w26
    "Status Control" <- w25
    n131 = Or(x=w31, y=w29) -> (x .or. y?=w30:bool)
  }
